vi "pulse.vi"(0 "VISA resource name":refnum<visa-resource-name>="COM1", 1 "Baud Rate":u32=115200, 2 "Data Bits":u16=8 min=5 max=8 step=1, 3 "Parity":u16(ring) items=["None", "Odd", "Even", "Mark", "Space"], 4 "Stop Bits":u16(ring)=10 items=["1.0"=10, "1.5"=15, "2.0"=20], 5 "Write & Read":bool=TRUE, 7 "Flow Control":u16(ring) items=["None"=0, "XON/XOFF"=1, "RTS/CTS"=2, "DTR/DSR"=4]) -> (9 "Read String":string, 10 "Bytes Read":u32)   [LabVIEW 2017]
doc: "The Basic Serial Read and Write example performs a Serial Port Read, a Serial Port Write, or a combination of these actions. The user selects the actions (read or write) on the front panel. If both are selected, the VI will write the data first, read data, and then close the VISA session that is opened to the port. This VI will wait until the specified number of bytes is received at the port. Only the number of bytes specified will be read.\n\nINSTRUCTIONS:\n1) Select the serial resource and configuration parameters (baud rate, data bits, parity, stop bits, flow control).\n2) Select the operations to be performed. \n3) Connect the serial port to your device. If no device is available, perform a loopback test by doing one of the following. Short pins 2 and 3 on a RS-232 cable or short pin 4 to pin 8 and pin 5 to pin 9 on a RS-485/422 cable. \n4) Run the VI to see the data read. (The \"read string\" will match the \"string to write\" if a loopback test was performed.)\n\nNote: The parameters set for the serial port must match the parameters of the connected instrument or device. In this example, the bytes to read parameter specifies the number of bytes that the serial port reads. If there were more bytes at the port than the number specified in bytes to read, those bytes would not be read. Also, if you specify to read more bytes than the number of bytes actually read, you might receive a timeout error message.\n\nOn the block diagram, the Configure Serial Port VI sets the configuration parameters. The front panel displays the controls used to configure the basic parameters, such as baud rate, data bits, and parity. Constants configure the other parameters the user probably does not need set. After the VISA Configure Serial Port VI opens the VISA session and configures the port, the VI passes the VISA resource name to other VIs that perform operations on that VISA resource. The VISA Write function sends a command to the serial device and the VISA Read function returns data based on the command. The VISA Close function then closes the reference to the serial device. It is important to close the reference; otherwise communication through with that port through protocols other than VISA might not be possible."
uses:
  <vilib>/Analysis/1siggen.llb/Ramp Pattern by Samples.vi
  <vilib>/Instr/_visa.llb/VISA Configure Serial Port (Instr).vi
  <vilib>/Utility/file.llb/Write Delimited Spreadsheet (DBL).vi
  <vilib>/ptbypt/NI_PtbyPt.lvlib
  <vilib>/Analysis/NI_AAL_SigProc.lvlib
  <vilib>/Analysis/NI_AALBase.lvlib
panel:
  out "Danger Level":bool
  out "BPM Meter":dbl(knob) scale=0.0..150.0
  out "BPM":dbl
  in  "?":bool
  in  "Stop Button":bool
  in  "LOAD":bool
  in  "SAVE":bool
  in  "Flow Control 2":u16(ring) items=["16"=16, "32"=32, "64"=64, "128"=128]
  out "1_index":dbl
  out "0_index":dbl
  out "valley 2":bool
  out "peak 2":bool
  in  "threshold 2":dbl(slide) scale=-15.0..15.0
  in  "peaks/valleys 2":enum32{"Peaks", "Valleys"}(ring)
  in  "width 2":i32(slide)=10 min=3 scale=3.0..20.0
  out "Signal Input and Peaks/Valleys from Peak Detector 2":cluster{"Locations":dbl[], "Amplitudes":dbl[]}[](graph)
  out "2nd Derivatives 2":dbl[](array[numeric])
  out "Amplitudes 2":dbl[](array[numeric])
  out "Locations 2":dbl[](array[numeric])
  out "# found 2":i32=4
  out "Waveform Chart":dbl(graph)
  in  "Apply":bool
  out "Load":cluster{"Y":dbl[], dbl[]}(graph)
  out "Current Reading":string
  out "Iterations / Sec.":dbl
  out "Elapsed Time (s)":dbl
  out "Iterations":i32
  in  "stop":bool
  in  "Delay Before Read (mS)":u32=50
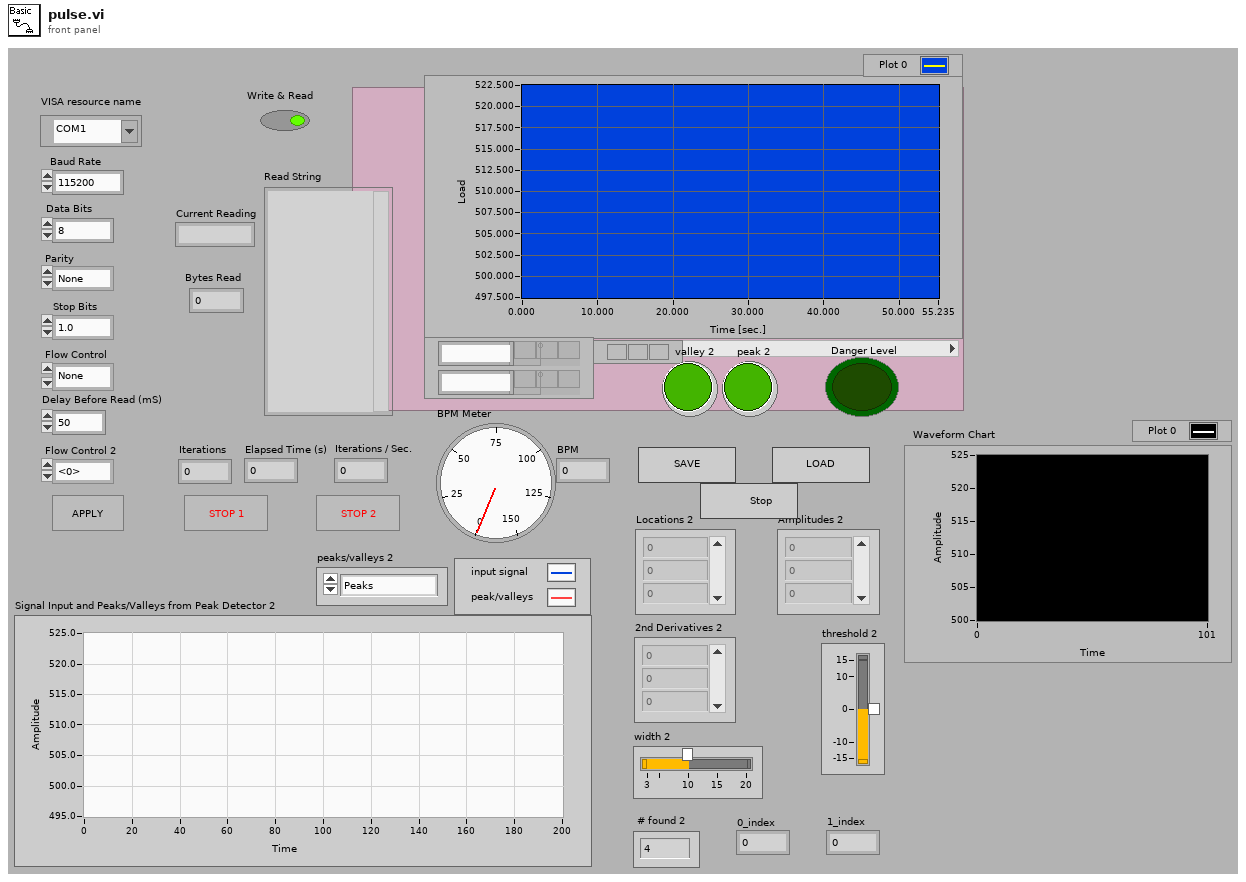
[diagram p1: front panel]
types:
  T1 = cluster{"Ramp Pattern":dbl[], "Current Queue":dbl[]}
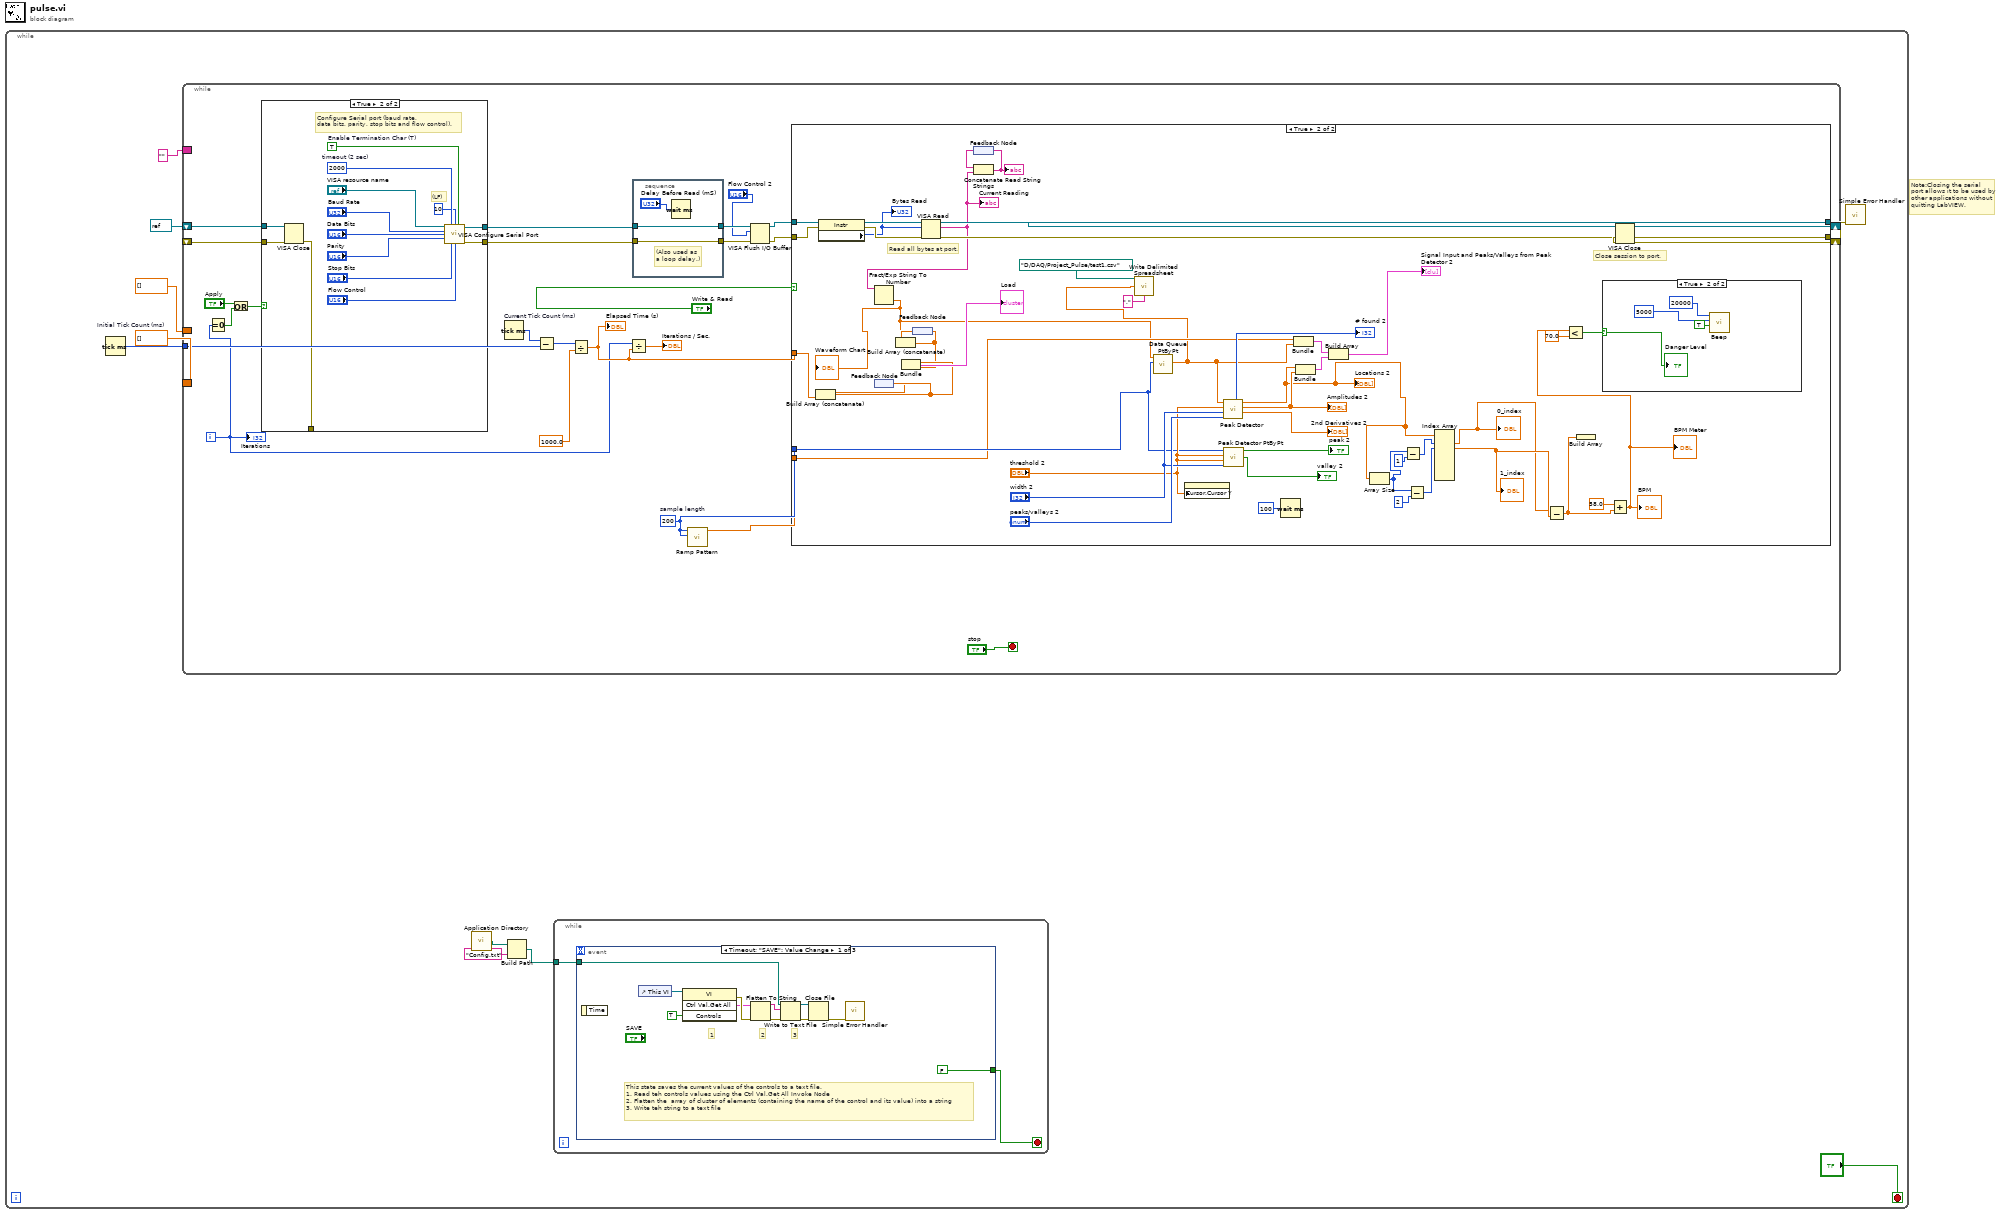
[diagram p0: block diagram]
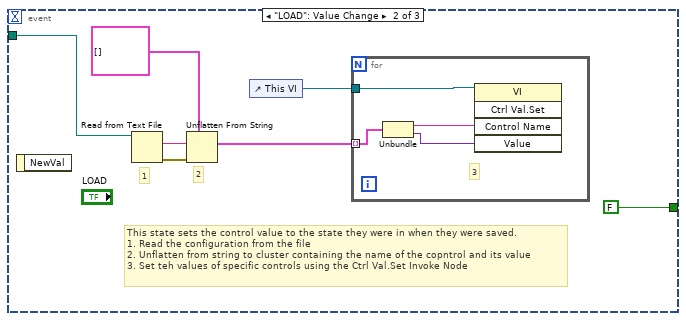
[diagram p2: hidden frame]
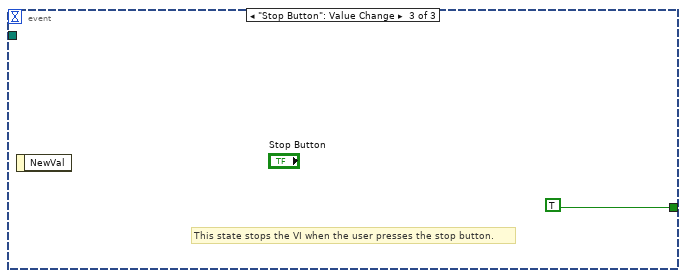
[diagram p3: hidden frame]
diagram:
  # "Note:Closing the serial port allows it to be used by other applications without\nquitting LabVIEW."
  n1 = while {
    stop <- "?" stop-if-true
    # "Close session to port."
    n2 = Tick Count (ms) "Initial Tick Count (ms)"() -> (millisecond timer value=w10:u32)
    n3 = while {
      tunnel: w10 -> [w56]
      border: "" -> [_]
      border: dbl[] [] -> [_]
      border: dbl[] [] -> [_]
      shift-right: [w61] -> w12
      shift-left: refnum<visa-resource-name> refnum ("VISA resource name out") -> [w52]
      shift-right: [w62] -> w11
      shift-left: _ -> [w51]
      i -> [w48]
      stop <- "stop" stop-if-true
      w46 = 200  # sample length
      n4 = Equal To 0?(x=w48) -> (x = 0?=w49:bool)
      n5 = Or(x="Apply", y=w49) -> (x .or. y?=w50:bool)
      n6 = case shown="True" w50 {
        tunnel: [w117 w123] -> w39
        tunnel: [w116 w122] -> w38
        tunnel: w52 -> [w117 w121]
        tunnel: w51 -> [w116 w120]
        tunnel: [_ w119] -> _
        frame False {
        }
        frame True {
          w127 = TRUE  # Enable Termination Char (T)
          w128 = u32 2000  # timeout (2 sec)
          # "(LF)"
          # "Configure Serial port (baud rate,\ndata bits, parity, stop bits and flow control)."
          n7 = VISA Close(VISA resource name=w121, error in (no error)=w120) -> (error out=w119:errorcluster)
          n8 = call-poly "VISA Configure Serial Port"("VISA resource name"="VISA resource name", "timeout (10sec)"=w128, "termination char\n(0xA = '\\n' = LF)"=u8 10 ("termination char\n(0xA = '\\n' = LF)"), "Enable Termination\nChar (T)"=w127, "baud rate (9600)"="Baud Rate", "data bits (8)"="Data Bits", "parity (0:none)"="Parity", "stop bits (10: 1 bit)"="Stop Bits", "flow control (0:none)"="Flow Control") -> ("VISA resource name out"=w123:refnum<visa-resource-name>, "error out"=w122:errorcluster)  [unwired: 5 in]
        }
      }
      n9 = Tick Count (ms) "Current Tick Count (ms)"() -> (millisecond timer value=w59:u32)
      n10 = Subtract(x=w59, y=w56) -> (x-y=w58:u32)
      n11 = Divide(x=w58, y=1000.0) -> (x/y=w54:dbl)
      "Elapsed Time (s)" <- w54
      n12 = Divide(x=w48, y=w54) -> (x/y=→"Iterations / Sec.":dbl)
      n13 = stacked-sequence {
        tunnel: w38 -> [w134]
        tunnel: [w134] -> w43
        tunnel: w39 -> [w133]
        tunnel: [w133] -> w44
        frame #0 {
          # "(Also used as\na loop delay.)"
          n14 = Wait (ms)(milliseconds to wait="Delay Before Read (mS)") -> ()  [unwired: 1 out]
        }
      }
      n15 = call-poly <vilib>:"Ramp Pattern.vi"("end"=w46, "samples"=w46) -> ("Ramp Pattern"=w45:dbl[])  [unwired: 8 in, 1 out]
      n16 = VISA Flush I/O Buffer(VISA resource name=w44, mask (16)="Flow Control 2", error in (no error)=w43) -> (VISA resource name out=w41:refnum<visa-resource-name>, error out=w42:errorcluster)
      n17 = case shown="True" "Write & Read" {
        tunnel: w42 -> [w63 w111]
        tunnel: w41 -> [w64 w110]
        tunnel: [w63 w109] -> w62
        tunnel: [w64 w108] -> w61
        tunnel: w54 -> [_ w101]
        tunnel: w46 -> [_ w84]
        tunnel: w45 -> [_ w83]
        frame False {
        }
        frame True {
          # "Read all bytes at port."
          n18 = property class="Instr"(reference=w110, error in=w111) -> (reference out=w107:refnum<visa-resource-name>, error out=w106:errorcluster, "Serial Settings:Number of Bytes at Serial Port"=w105:u32)
          "Bytes Read" <- w105
          n19 = feedback #1() -> (w98:dbl[])
          n20 = Build Array (concatenate)(w98, w101) -> (w99:dbl[])
          n21 = feedback-in #1(w99) -> ()
          n22 = feedback #2() -> (w96:dbl[])
          n23 = VISA Read(VISA resource name=w107, byte count=w105, error in (no error)=w106) -> (VISA resource name out=w108:refnum<visa-resource-name>, read buffer=w102:string, error out=w109:errorcluster)  [unwired: 1 out]
          "Current Reading" <- w102
          n24 = Fract/Exp String To Number(string=w102) -> (number=w71:dbl)  [unwired: 3 in, 1 out]
          "Waveform Chart" <- w71
          n25 = Build Array (concatenate)(w96, w71) -> (w97:dbl[])
          n26 = Bundle(w99, w97) -> (→"Load":cluster{dbl[], dbl[]})  [unwired: 1 in]
          n27 = feedback-in #2(w97) -> ()
          n28 = feedback #3() -> (w103:string)
          n29 = Concatenate Strings(w103, w102) -> (w104:string)
          "Read String" <- w104
          n30 = feedback-in #3(w104) -> ()
          n31 = call <vilib>:"Data Queue PtByPt.vi"("sample length"=w84, "input data point"=w71) -> ("Current Queue"=w68:dbl[])  [unwired: 5 in, 4 out]
          n32 = call-poly <vilib>:"Write Delimited Spreadsheet.vi"("file path (dialog if empty)"=path "D:/DAQ/Project_Pulse/test1.csv", "1D data"=w68, "delimiter (\\t)"="," ("delimiter (\\t)")) -> ()  [unwired: 11 in, 2 out]
          n33 = property on="Signal Input and Peaks/Valleys from Peak Detector 2" class="XYGraph (strict)"("Cursor.Cursor Y"="threshold 2") -> ()  [unwired: 2 in, 2 out]
          n34 = call <vilib>:"Peak Detector.vi"("peaks/valleys"="peaks/valleys 2", "width"="width 2", "threshold"="threshold 2", "X"=w68) -> ("2nd Derivatives"=→"2nd Derivatives 2":dbl[], "Amplitudes"=w89:dbl[], "Locations"=w76:dbl[], "# found"=→"# found 2":i32)  [unwired: 3 in, 1 out]
          "Locations 2" <- w76
          "Amplitudes 2" <- w89
          n35 = call <vilib>:"Peak Detector PtByPt.vi"("x"=w84, "threshold peak"="threshold 2", "threshold valley"="threshold 2", "width"="width 2") -> ("peak"=→"peak 2":bool, "valley"=→"valley 2":bool)  [unwired: 1 in, 1 out]
          n36 = Wait (ms)(milliseconds to wait=u32 100) -> ()  [unwired: 1 out]
          n37 = Bundle("Ramp Pattern"=w83, "Current Queue"=w68) -> (w94:T1)  [unwired: 1 out]
          n38 = Bundle("Locations"=w76, "Amplitudes"=w89) -> (w92:cluster{"Locations":dbl[], "Amplitudes":dbl[]})  [unwired: 1 out]
          n39 = Build Array(w94, w92) -> (→"Signal Input and Peaks/Valleys from Peak Detector 2":cluster{"Locations":dbl[], "Amplitudes":dbl[]}[])
          n40 = Array Size(array=w76) -> (size(s)=w77:i32)
          n41 = Subtract(x=w77, y=1) -> (x-y=w80:i32)
          n42 = Subtract(x=w77, y=2) -> (x-y=w78:i32)
          n43 = Index Array(array=w76, index #1=w80, index #2=w78) -> (element #1=w74:dbl, element #2=w75:dbl)  [unwired: 6 in, 6 out]
          "0_index" <- w74
          "1_index" <- w75
          n44 = Subtract(x=w74, y=w75) -> (x-y=w73:dbl)
          n45 = Build Array(w73) -> ()  [unwired: 1 out]
          n46 = Add(x=58.0, y=w73) -> (x+y=w66:dbl)
          "BPM" <- w66
          "BPM Meter" <- w66
          n47 = Less?(x=w66, y=70.0) -> (x < y?=w67:bool)
          n48 = case shown="True" w67 {
            selector: w67 -> [_ w112]
            frame False {
            }
            frame True {
              n49 = call <vilib>:"Beep.vi"("use system alert? (T)"=TRUE, "duration (msec)"=u32 5000, "frequency (Hz)"=u32 20000) -> ()  [unwired: 9 in]
              "Danger Level" <- w112
            }
          }
        }
      }
      "Iterations" <- w48
    }
    n50 = call <vilib>:"Application Directory.vi"() -> ("Application Directory"=w5:path)
    n51 = Build Path(base path=w5, name or relative path="Config.txt") -> (appended path=w3:path)
    n52 = while {
      tunnel: w3 -> [w13]
      stop <- w14 stop-if-true
      n53 = event shown="[0] Timeout;  \"SAVE\": Value Change" {
        selector: _ -> [_ _ _]
        dyn-events: _ -> [_ _ _]
        timeout: _ -> [_ _ _]
        tunnel: [FALSE FALSE TRUE] -> w14
        tunnel: w13 -> [w15 w26 _]
        event Timeout; "SAVE": Value Change {
          # "3"
          # "2"
          # "1"
          # "This state saves the current values of the controls to a text file.\n1. Read teh controls values using the Ctrl Val.Get All Invoke Node\n2. Flatten the  array of cluster of elements (containing the name of the control and its value) into a string\n3. Write teh string to a text file"
          n54 = event-data() -> ()  [unwired: 1 in, 1 out]
          n55 = control-ref of="This VI"() -> (w25:refnum<vi>)
          n56 = invoke class="VI" method="Ctrl Val.Get All"(reference=w25, "Controls"=TRUE) -> (error out=w21:errorcluster, "Get All Control Values Variant"=w20:cluster{"Name":string, "Variant Data":variant}[])  [unwired: 2 in, 2 out]
          n57 = Flatten To String(anything=w20, error in (no error)=w21) -> (data string=w22:string, error out=w23:errorcluster)  [unwired: 2 in, 1 out]
          n58 = Write to Text File(file (use dialog)=w15, text=w22, error in=w23) -> (refnum out=w18:refnum<file>, error out=w19:errorcluster)  [unwired: 1 in, 1 out]
          n59 = Close File(refnum=w18, error in=w19) -> (error out=w17:errorcluster)  [unwired: 1 out]
          n60 = call <vilib>:"Simple Error Handler.vi"("error in (no error)"=w17) -> ()  [unwired: 4 in, 5 out]
        }
        event "LOAD": Value Change {
          # "2"
          # "1"
          # "This state sets the control value to the state they were in when they were saved.\n1. Read the configuration from the file\n2. Unflatten from string to cluster containing the name of the copntrol and its value\n3. Set teh values of specific controls using the Ctrl Val.Set Invoke Node"
          n61 = event-data() -> ()  [unwired: 1 in, 1 out]
          n62 = Read from Text File(file (use dialog)=w26) -> (text=w30:string, error out=w31:errorcluster)  [unwired: 3 in, 2 out]
          n63 = Unflatten From String(type=cluster{string, variant}[] [], binary string=w30, error in (no error)=w31) -> (value=w28:cluster{string, variant}[])  [unwired: 2 in, 2 out]
          n64 = control-ref of="This VI"() -> (w29:refnum<vi>)
          n65 = for {
            tunnel: w29 -> [w36]
            tunnel: w28 -> [w35] mode=indexing
            # "3"
            n66 = Unbundle(w35) -> (w33:string, w34:variant)
            n67 = invoke class="VI" method="Ctrl Val.Set"(reference=w36, "Control Name"=w33, "Value"=w34) -> ()  [unwired: 2 in, 5 out]
          }
        }
        event "Stop Button": Value Change {
          # "This state stops the VI when the user presses the stop button."
          n68 = event-data() -> ()  [unwired: 1 in, 1 out]
        }
      }
    }
    n69 = VISA Close(VISA resource name=w12, error in (no error)=w11) -> (error out=w1:errorcluster)
    n70 = call <vilib>:"Simple Error Handler.vi"("error in (no error)"=w1) -> ()  [unwired: 4 in, 5 out]
  }
